vi "Switch mode for pco.edge.vi"() -> ()   [LabVIEW 2012]
doc: "A very basic example of how to switch the shutter mode of the pco.edge. Select the desired shutter mode before running the VI."
panel:
  in  "Shutter mode: set this before running VI":u32(ring)=1 items=["Rolling shutter"=1, "Global shutter"=2]
  in  "Timeouts (ms)":u32[](array[numeric])=[2000, 3000, 250]
  out "Name":string
  # "Switch mode: This VI will set the shutter mode, reboot, wait 10 seconds then read the camera name to verify the change"
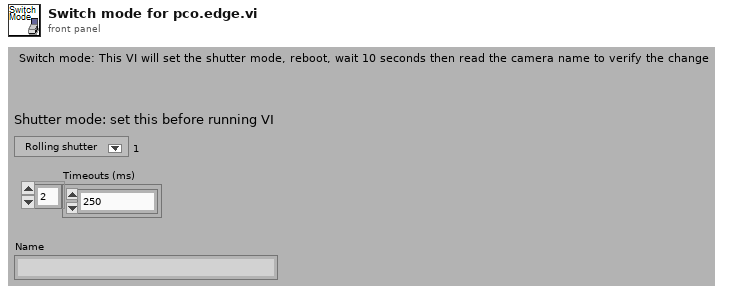
[diagram p1: front panel]
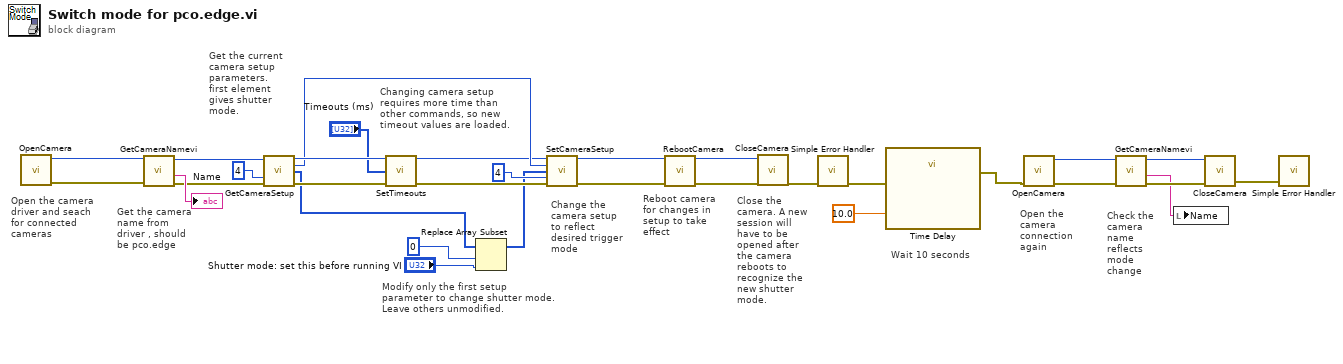
[diagram p0: block diagram]
diagram:
  # "Check the camera name reflects mode change"
  # "Open the camera connection again"
  # "Wait 10 seconds"
  # "Close the camera. A new session will have to be opened after the camera reboots to recognize the new shutter mode."
  # "Reboot camera for changes in setup to take effect"
  # "Change the camera setup to reflect desired trigger mode"
  # "Changing camera setup requires more time than other commands, so new timeout values are loaded."
  # "Modify only the first setup parameter to change shutter mode. Leave others unmodified."
  # "Get the current camera setup parameters. first element gives shutter mode."
  # "Get the camera name from driver , should be pco.edge"
  # "Open the camera driver and seach for connected cameras"
  n1 = call "OpenCamera.vi"() -> ("ErrorOut"=w15:errorcluster, "Handle out"=w17:u64)  [unwired: 4 in, 2 out]
  n2 = call "GetCameraNamevi.vi"("ErrorIn"=w15, "Handle in"=w17) -> ("ErrorOut"=w14:errorcluster, "Name"=→"Name":string, "Handle out"=w16:u64)  [unwired: 6 in, 1 out]
  n3 = call "GetCameraSetup.vi"("ph"=w16, "Len"=u16 4, "error in (no error)"=w14) -> ("hout"=w27:u64, "Type"=w24:u16, "Setup"=w12:u32[], "error out"=w26:errorcluster)  [unwired: 8 in, 1 out]
  n4 = call "SetTimeouts.vi"("ph"=w27, "Timeouts (ms)"="Timeouts (ms)", "error in (no error)"=w26) -> ("hout"=w19:u64, "error out"=w18:errorcluster)  [unwired: 10 in, 1 out]
  n5 = Replace Array Subset(array=w12, new element="Shutter mode: set this before running VI", index=0) -> (w10:u32[])
  n6 = call "SetCameraSetup.vi"("ph"=w19, "Type"=w24, "Setup"=w10, "Len"=u16 4, "error in (no error)"=w18) -> ("hout"=w22:u64, "error out"=w21:errorcluster)  [unwired: 8 in, 1 out]
  n7 = call "RebootCamera.vi"("ph"=w22, "error in (no error)"=w21) -> ("hout"=w29:u64, "error out"=w28:errorcluster)  [unwired: 11 in, 1 out]
  n8 = call "CloseCamera.vi"("ErrorIn"=w28, "Handle in"=w29) -> ("ErrorOut"=w20:errorcluster)  [unwired: 1 in, 2 out]
  n9 = call <vilib>:"Simple Error Handler.vi"("error in (no error)"=w20) -> ("error out"=w9:errorcluster)  [unwired: 4 in, 4 out]
  n10 = call "Time Delay"("error in (no error)"=w9, "Delay Time (s)"=10.0) -> ("error out"=w7:errorcluster)  [unwired: 9 in]
  n11 = call "OpenCamera.vi"("ErrorIn"=w7) -> ("ErrorOut"=w6:errorcluster, "Handle out"=w5:u64)  [unwired: 3 in, 2 out]
  n12 = call "GetCameraNamevi.vi"("ErrorIn"=w6, "Handle in"=w5) -> ("ErrorOut"=w4:errorcluster, "Name"=w1:string, "Handle out"=w3:u64)  [unwired: 6 in, 1 out]
  n13 = local write "Name"(w1) -> ()
  n14 = call "CloseCamera.vi"("ErrorIn"=w4, "Handle in"=w3) -> ("ErrorOut"=w2:errorcluster)  [unwired: 1 in, 2 out]
  n15 = call <vilib>:"Simple Error Handler.vi"("error in (no error)"=w2) -> ()  [unwired: 4 in, 5 out]
